vi "Mux16.vi"(3 "sel":bool, 6 "b":bool[](array[boolean]), 7 "a":bool[](array[boolean])) -> (1 "out":bool[](array[boolean]))   [LabVIEW 2014]
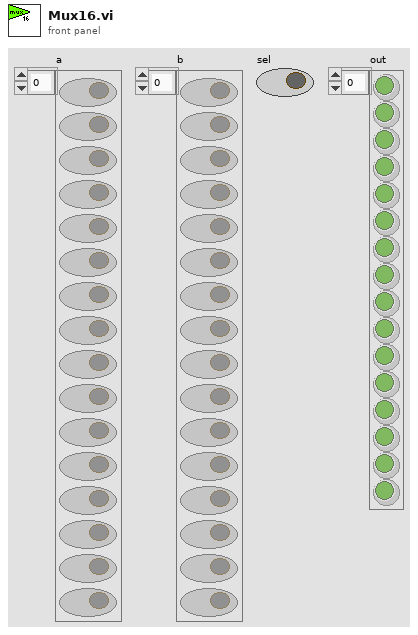
[diagram p1: front panel]
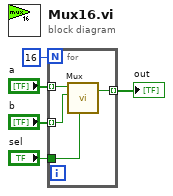
[diagram p0: block diagram]
diagram:
  n1 = for {
    N: 16 -> [_]
    tunnel: "a" -> [w9] mode=indexing
    tunnel: "b" -> [w8] mode=indexing
    tunnel: [w6] -> w2 mode=indexing
    tunnel: "sel" -> [w7]
    n2 = call "Mux.vi"("sel"=w7, "b"=w8, "a"=w9) -> ("out"=w6:bool)  [unwired: 4 in]
  }
  "out" <- w2
